vi "Set Array Control Enabled State.vi"(7 "enabled (T)":bool=TRUE, 10 "error in (no error)":errorcluster, 11 "reference array in":refnum<vi>[](array[refnum])) -> (2 "error out":errorcluster, 3 "reference array out":refnum<vi>[](array[refnum]))   [LabVIEW 2020, in "varilib.lvlib"]
doc: "Change enabled state of the array of referenced controls to 'Enabled' or 'Disabled and Grayed Out'. The status of the error in input is not important."
uses:
  varilib.lvlib
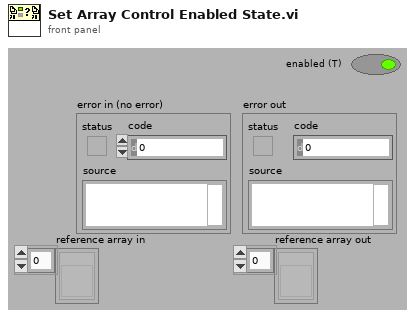
[diagram p1: front panel]
types:
  T1 = enum8{"Enabled", "Disabled", "Disabled and Grayed Out"}
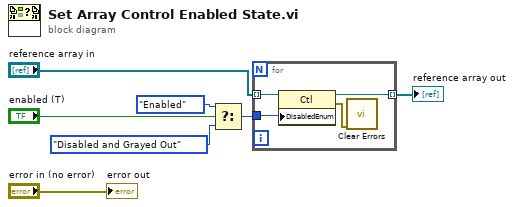
[diagram p0: block diagram]
diagram:
  n1 = Select(t=T1."Enabled" ("Disabled"), s="enabled (T)", f=T1."Disabled and Grayed Out" ("Disabled")) -> (s? t:f=w7:T1)
  n2 = for {
    tunnel: w7 -> [w11]
    tunnel: "reference array in" -> [w9] mode=indexing
    tunnel: [w8] -> w1 mode=indexing
    n3 = property class="Ctl"(reference=w9, "DisabledEnum"=w11) -> (reference out=w8:refnum<vi>, error out=w10:errorcluster)  [unwired: 1 in]
    n4 = call <vilib>:"Clear Errors.vi"("error in (no error)"=w10) -> ()  [unwired: 5 in, 2 out]
  }
  "reference array out" <- w1
  "error out" <- "error in (no error)"
